vi "Remote Video snapshot.vi"(1 "Quality":u32=750 max=1000, 2 "Resolution":T1=1 items=["Low", "Med", "High", "Max."], 3 "Camera":T2="Travcam") -> (0 "Error out":errorcluster)   [LabVIEW 2015]
uses:
  Camera enum/Camera enum.ctl
  Camera enum/Camera resolution.ctl
  Globals/CamServer global.vi
panel:
  # "PN 27/08/15"
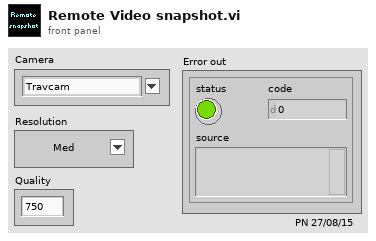
[diagram p1: front panel]
types:
  T1 = typedef "Camera resolution.ctl" = u8
  T2 = typedef "Camera enum.ctl" = string
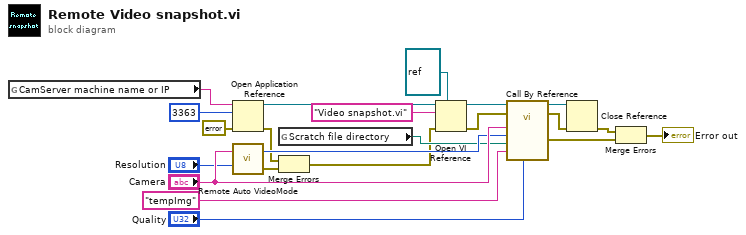
[diagram p0: block diagram]
diagram:
  n1 = global read "CamServer global.vi" "CamServer machine name or IP"() -> (w7:string)
  n2 = Open Application Reference(8:errorcluster {"status"=FALSE, "code"=0, "source"=""} ("error in (no error)"), 10:u16 3363 ("port"), 11:w7) -> (0:w5:errorcluster, 3:w20:refnum<vi>)  [unwired: 1 in]
  n3 = call "Remote Auto VideoMode.vi"("Resolution"="Resolution", "Camera"="Camera") -> ("Error out"=w4:errorcluster, "VideoMode"=w10:u32)
  n4 = global read "CamServer global.vi" "Scratch file directory"() -> (w6:path)
  n5 = Merge Errors(w5, w4) -> (w3:errorcluster)
  n6 = Open VI Reference(type specifier VI Refnum (for type only)=refnum<vi> refnum, application reference (local)=w20, vi path="Video snapshot.vi" ("machine name"), error in (no error)=w3) -> (vi reference=w18:refnum<vi>, error out=w19:errorcluster)  [unwired: 2 in]
  n7 = call-by-ref "?"(reference=w18, error in=w19, "Quality"="Quality", "Image name"="tempImg", "Image directory path"=w6, "VideoMode"=w10, "Interface name"="Camera") -> (reference out=w16:refnum<vi>, error out=w15:errorcluster, "Error Out"=w14:errorcluster)  [unwired: 1 in]
  n8 = Close Reference(reference=w16, error in (no error)=w15) -> (error out=w13:errorcluster)
  n9 = Merge Errors(w13, w14) -> (→"Error out":errorcluster)
